vi "BPSK_Sync.vi"(4 "UpSampleRate":dbl, 6 "data":dbl[](array[numeric]), 7 "Preamble":dbl[](array[numeric]), 8 "error in (no error)":errorcluster caption="错误输入（无错误）", 10 "input_data":dbl[](array[numeric]) format="%#_13g", 11 "PathIn":path) -> (0 "error out":errorcluster caption="错误输出", 2 "output_data":dbl[](array[numeric]), 3 "PathOut":path, 5 "RecvCorr":dbl[](array[numeric]))   [LabVIEW 2015]
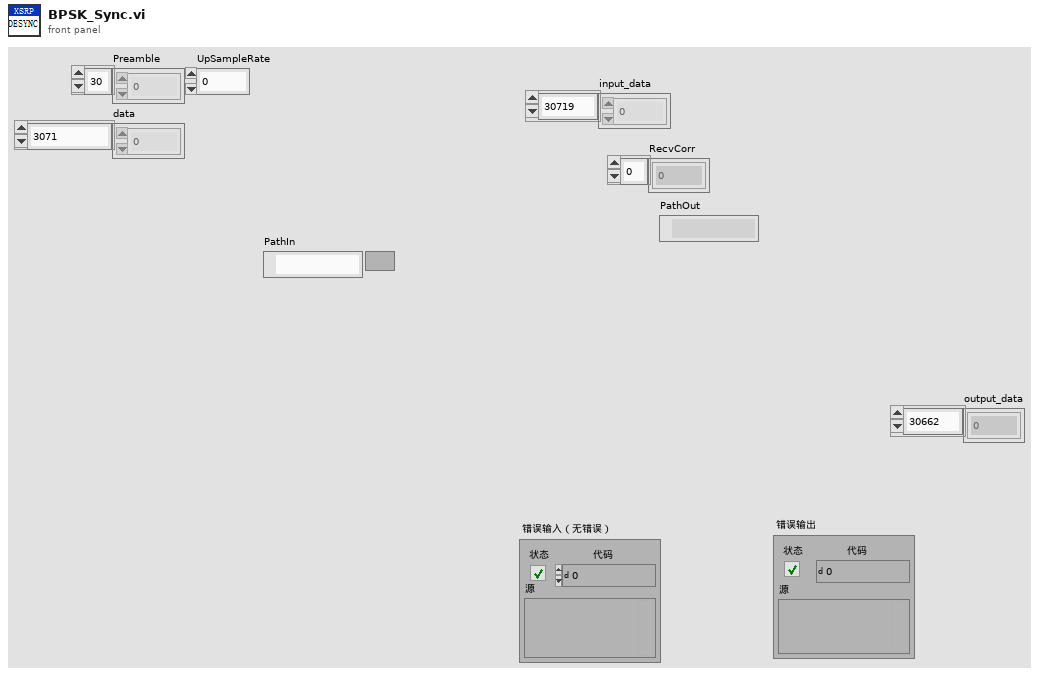
[diagram p1: front panel]
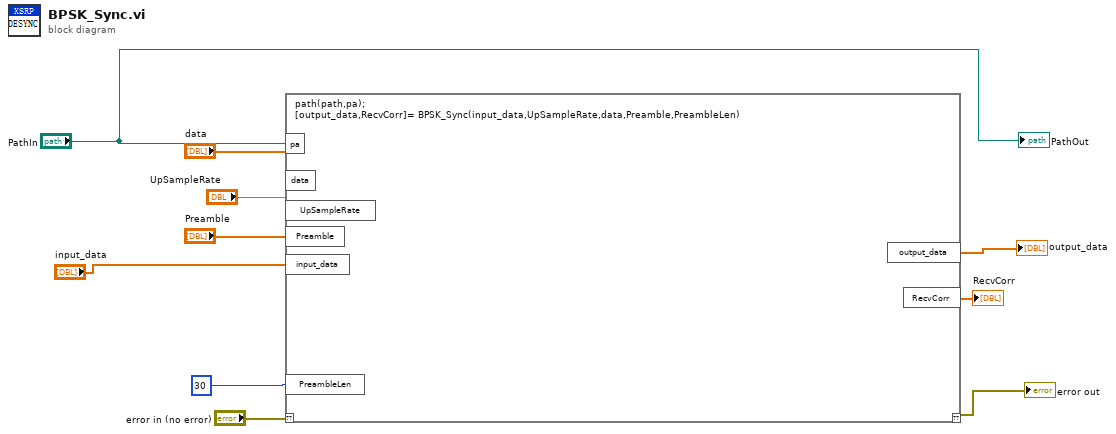
[diagram p0: block diagram]
diagram:
  n1 = script code="path(path,pa);\n[output_data,RecvCorr]= BPSK_Sync(input_data,UpSampleRate,data,Preamble,PreambleLen)"("??"="error in (no error)", "pa"="PathIn", "input_data"="input_data", "UpSampleRate"="UpSampleRate", "data"="data", "Preamble"="Preamble", "PreambleLen"=30) -> ("??"=→"error out":errorcluster, "output_data"=→"output_data":dbl[], "RecvCorr"=→"RecvCorr":dbl[])
  "PathOut" <- "PathIn"
